vi "New motor Control integrated remodeled (main).vi"(0 "States":enum16{"RESET ENCODER", "WRITE", "READ", "INIT"}(ring), 1 "Target Speed":T2 {"wTargetSpeed" scale=-1.0..1.0; "yTargetSpeed" scale=-1.0..1.0; "xTargetSpeed" scale=-1.0..1.0}, 3 "Error in":errorcluster, 4 "Boolean":bool=TRUE) -> (5 "Speed and distance cluster":T1, 6 "Error out":errorcluster)   [LabVIEW 2018]
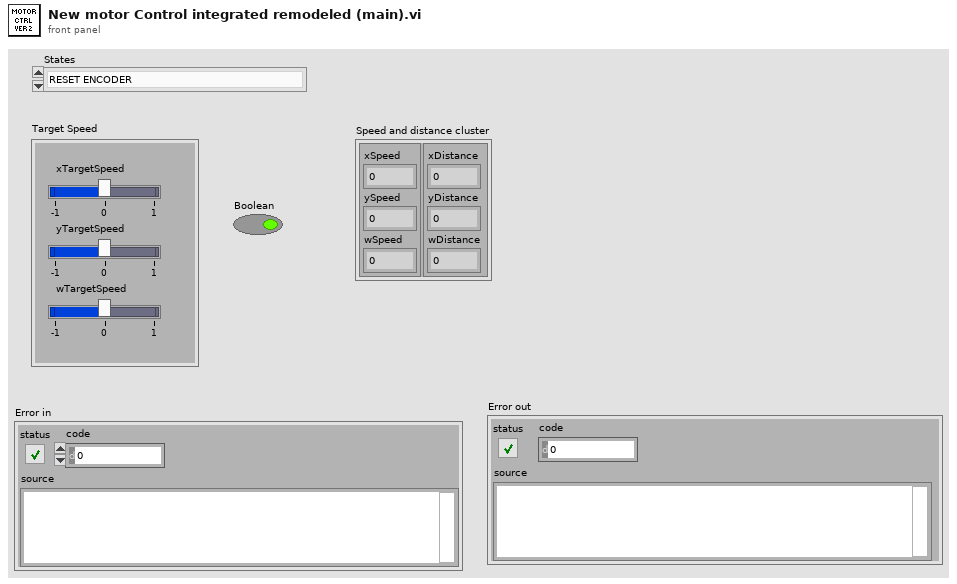
[diagram p1: front panel]
types:
  T1 = cluster{cluster{"xSpeed":dbl, "ySpeed":dbl, "wSpeed":dbl}, cluster{"xDistance":dbl, "yDistance":dbl, "wDistance":dbl}}
  T2 = cluster{"xTargetSpeed":dbl, "yTargetSpeed":dbl, "wTargetSpeed":dbl}
  T3 = cluster{"Encoder 0":dbl, "Encoder 1":dbl, "Encoder 2":dbl}
  T4 = cluster{"Distance M0 ":dbl, "Distance M1 ":dbl, "Distance M2 ":dbl}
  T5 = cluster{"xDistance":dbl, "yDistance":dbl, "wDistance":dbl}
  T6 = cluster{"xSpeed":dbl, "ySpeed":dbl, "wSpeed":dbl}
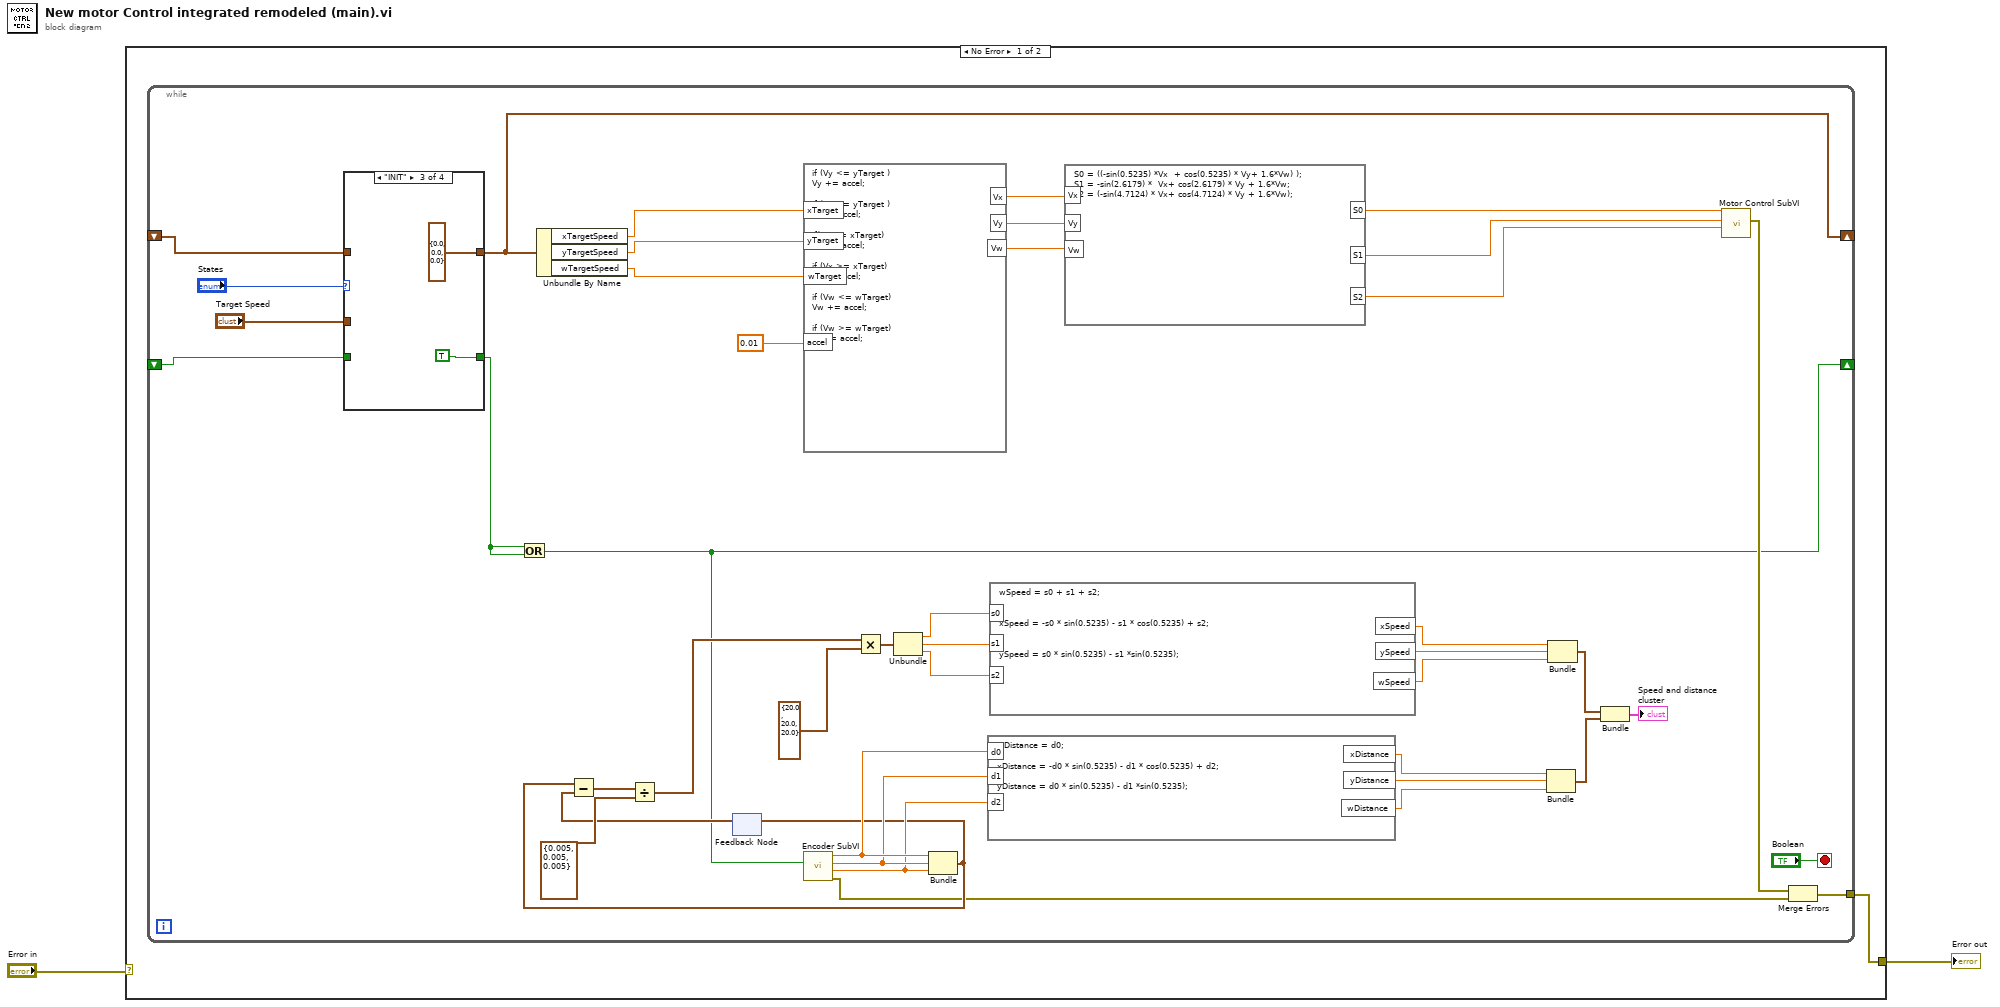
[diagram p0: block diagram]
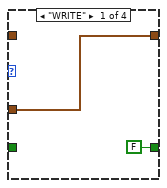
[diagram p2: hidden frame]
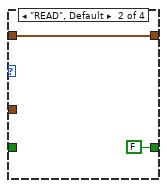
[diagram p3: hidden frame]
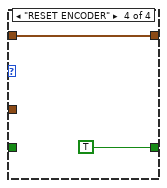
[diagram p4: hidden frame]
diagram:
  n1 = case shown="No Error" "Error in" {
    selector: "Error in" -> [_ w55]
    tunnel: [w3 w55] -> w1
    frame No Error {
      n2 = while {
        shift-right: [w25] -> _
        shift-left: _ -> [w24]
        tunnel: [w19] -> w3
        shift-right: [w18] -> _
        shift-left: _ -> [w16]
        stop <- "Boolean" stop-if-true
        n3 = case shown="\"INIT\"" "States" {
          tunnel: "Target Speed" -> [w48 _ _ _]
          tunnel: [w48 w50 T2 {"xTargetSpeed"=0.0, "yTargetSpeed"=0.0, "wTargetSpeed"=0.0} ("Target Speed") w54] -> w25
          tunnel: w24 -> [_ w50 _ w54]
          tunnel: [FALSE ("Reset Encoders") FALSE ("Reset Encoders") TRUE TRUE ("Reset Encoders")] -> w17
          tunnel: w16 -> [_ _ _ _]
          frame "WRITE" {
          }
          frame "READ", Default {
          }
          frame "INIT" {
          }
          frame "RESET ENCODER" {
          }
        }
        n4 = Or(x=w17, y=w17) -> (x .or. y?=w18:bool)
        n5 = Unbundle By Name(w25) -> ("xTargetSpeed"=w6:dbl, "yTargetSpeed"=w5:dbl, "wTargetSpeed"=w4:dbl)
        n6 = feedback #1() -> (w39:T4)  [unwired: 1 in]
        n7 = formula code="if (Vy <= yTarget )\nVy += accel;\n\nif (Vy >= yTarget )\nVy -= accel;\n\nif(Vx <= xTarget)\nVx += accel;\n\nif (Vx >= xTarget)\nVx -= accel;\n\nif (Vw <= wTarget)\nVw += accel;\n\nif (Vw >= wTarget)\nVw -= accel;"("xTarget"=w6, "yTarget"=w5, "wTarget"=w4, "accel"=0.01 ("input variable")) -> ("Vy"=w9:dbl, "Vx"=w10:dbl, "Vw"=w8:dbl)
        n8 = call "Encoder SubVI.vi"("Reset Encoders"=w18) -> ("error out"=w21:errorcluster, "Distance M2"=w36:dbl, "Distance M1"=w37:dbl, "Distance M0"=w38:dbl)  [unwired: 7 in]
        n9 = Bundle("Distance M0"=w38, "Distance M1"=w37, "Distance M2"=w36) -> (w28:T4)  [unwired: 1 in]
        n10 = Subtract(x=w28, y=w39) -> (x-y=w46:T4)
        n11 = Divide(x=w46, y=T3 {"Encoder 0"=0.005, "Encoder 1"=0.005, "Encoder 2"=0.005}) -> (x/y=w32:cluster{dbl, dbl, dbl})
        n12 = feedback-in #1(w28) -> ()
        n13 = Multiply(x=w32, y=cluster{dbl, dbl, dbl} {20.0, 20.0, 20.0}) -> (x*y=w15:cluster{dbl, dbl, dbl})
        n14 = Unbundle(w15) -> (w30:dbl, w41:dbl, w40:dbl)
        n15 = formula code="wDistance = d0;\n\nxDistance = -d0 * sin(0.5235) - d1 * cos(0.5235) + d2;\n\nyDistance = d0 * sin(0.5235) - d1 *sin(0.5235);"("d0"=w38, "d1"=w37, "d2"=w36) -> ("xDistance"=w35:dbl, "wDistance"=w33:dbl, "yDistance"=w34:dbl)
        n16 = formula code="wSpeed = s0 + s1 + s2;\n\n\nxSpeed = -s0 * sin(0.5235) - s1 * cos(0.5235) + s2;\n\n\nySpeed = s0 * sin(0.5235) - s1 *sin(0.5235);"("s0"=w30, "s1"=w41, "s2"=w40) -> ("xSpeed"=w43:dbl, "ySpeed"=w44:dbl, "wSpeed"=w42:dbl)
        n17 = formula code="S0 = ((-sin(0.5235) *Vx  + cos(0.5235) * Vy+ 1.6*Vw) );\nS1 = -sin(2.6179) *  Vx+ cos(2.6179) * Vy + 1.6*Vw;\nS2 = (-sin(4.7124) * Vx+ cos(4.7124) * Vy + 1.6*Vw);"("Vx"=w10, "Vy"=w9, "Vw"=w8) -> ("S0"=w14:dbl, "S1"=w13:dbl, "S2"=w12:dbl)
        n18 = Bundle("xDistance"=w35, "yDistance"=w34, "wDistance"=w33) -> (w23:T5)  [unwired: 1 in]
        n19 = Bundle("xSpeed"=w43, "ySpeed"=w44, "wSpeed"=w42) -> (w11:T6)  [unwired: 1 in]
        n20 = Bundle(w11, w23) -> (→"Speed and distance cluster":T1)  [unwired: 1 in]
        n21 = call "Motor Control SubVI.vi"("Speed M2"=w12, "Speed M1"=w13, "Speed M0"=w14) -> ("Motor Error"=w20:errorcluster)  [unwired: 8 in]
        n22 = Merge Errors(w20, w21) -> (w19:errorcluster)
      }
    }
    frame Error {
    }
  }
  "Error out" <- w1
